vi "doOperation.vi"(8 "error in (no error)":errorcluster, 9 "num2":dbl, 10 "num1":dbl, 11 "OperationAdd in":refnum<class "OperationAdd.lvclass">) -> (0 "error out":errorcluster, 3 "OperationAdd out":refnum<class "OperationAdd.lvclass">)   [LabVIEW 2017, in "OperationAdd.lvclass"]
uses:
  OperationAdd.lvclass
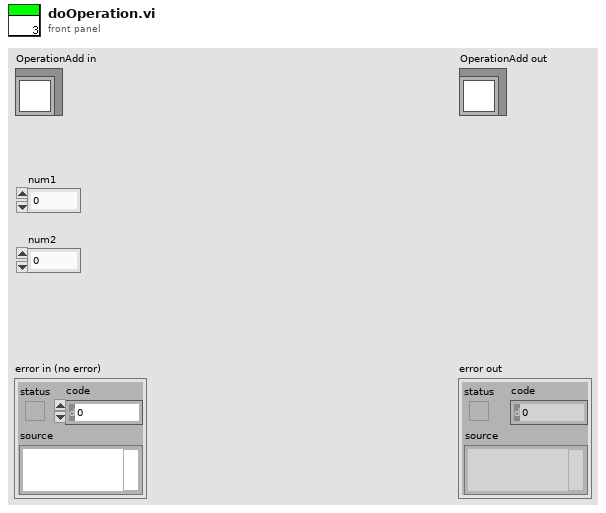
[diagram p1: front panel]
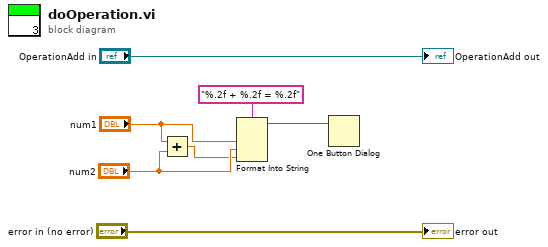
[diagram p0: block diagram]
diagram:
  n1 = Add(x="num1", y="num2") -> (x+y=w2:dbl)
  n2 = Format Into String(format string="%.2f + %.2f = %.2f", "num1", "num2", w2) -> (resulting string=w1:string)  [unwired: 2 in, 1 out]
  n3 = One Button Dialog(message=w1) -> ()  [unwired: 1 in, 1 out]
  "error out" <- "error in (no error)"
  "OperationAdd out" <- "OperationAdd in"
